vi "Cleanup.vi"(8 "error in":errorcluster, 11 "Philips Dialog in":refnum<class "Flex UI Dialog.lvclass">) -> (0 "error out":errorcluster)   [LabVIEW 2014, in "Flex UI Dialog.lvclass"]
doc: "Cleans up after the UI.\n\nRuns EVEN IF an error has occurred upstream."
uses:
  Flex UI Dialog.lvclass
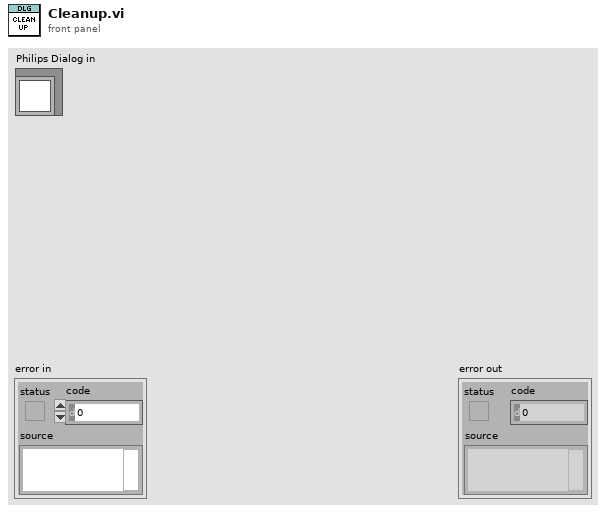
[diagram p1: front panel]
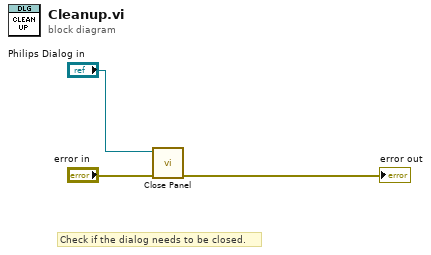
[diagram p0: block diagram]
diagram:
  # "Check if the dialog needs to be closed."
  n1 = call-dynamic "Close Panel.vi"("error in"="error in", "Philips Dialog in"="Philips Dialog in") -> ("error out"=→"error out":errorcluster)  [unwired: 8 in, 1 out]
